vi "graph4.vi"(11 "replay":bool) -> (0 "y":dynamicdata(graph), 3 "x":dynamicdata(graph), 4 "size(s)":i32)   [LabVIEW 2015]
uses:
  G_SEN.vi
  G_LCM.vi
  <vilib>/Analysis/polynomials.llb/1D Polynomial Evaluation (DBL).vi
  G_ALL.vi
  <vilib>/Analysis/NI_AALPro.lvlib
panel:
  out "y 4":dbl[](array[numeric])
  out "x 3":dbl[](array[numeric])
  out "y 3":dbl[](array[numeric])
  out "x 2":dbl[](array[numeric])
  in  "y 2":dbl=3.9000000000000004 format="%#_13g"
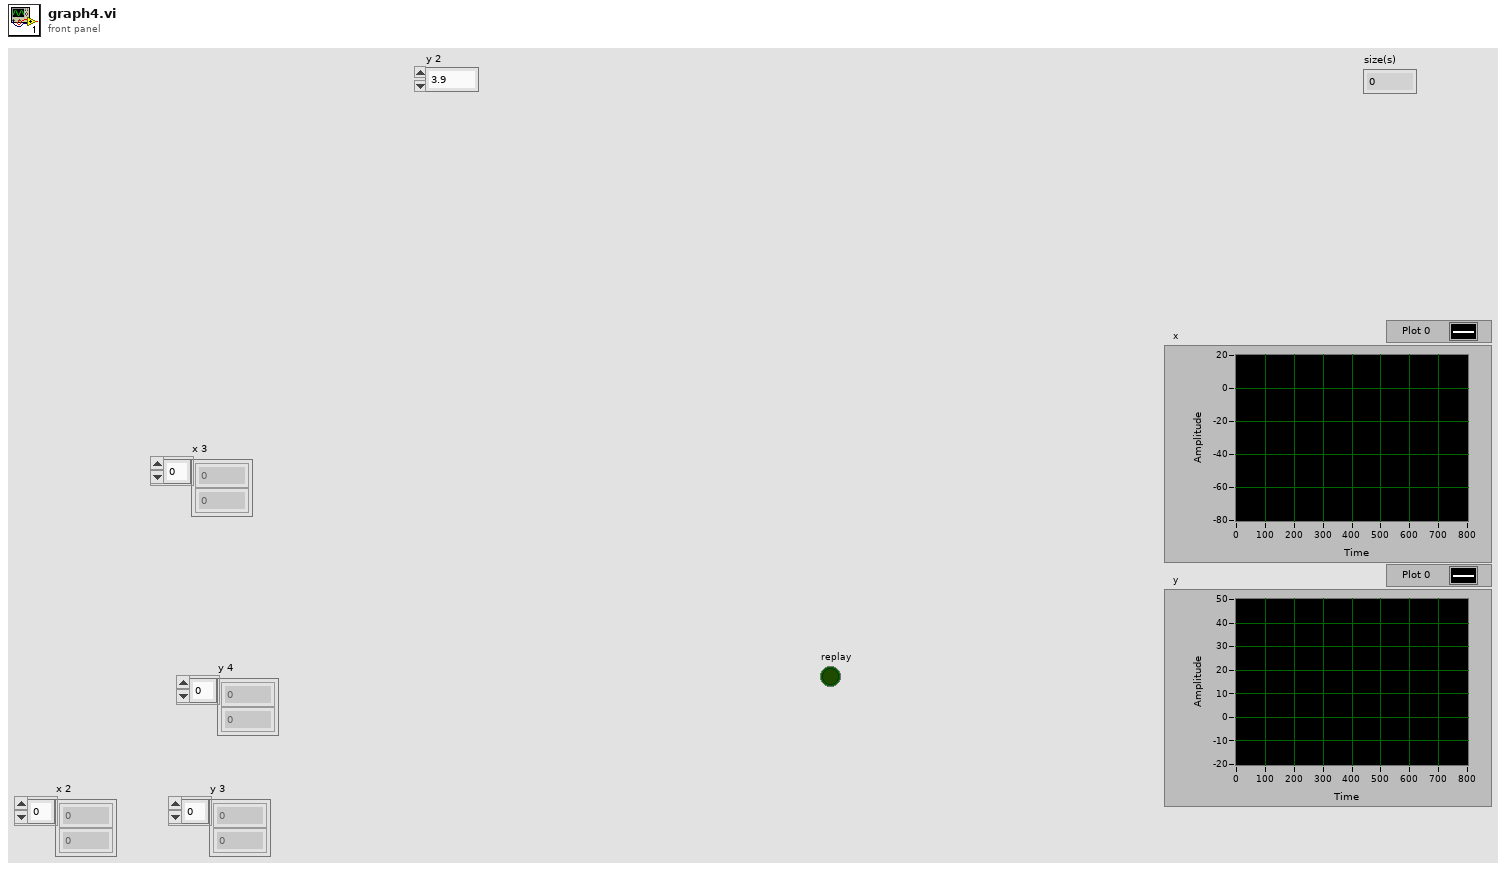
[diagram p1: front panel]
types:
  T1 = cluster{"Steer_input":dbl, "Steer_output":dbl, "VS_des":dbl, "VS_can":dbl, "heading":dbl, "auto":bool, "run":bool, "x":dbl, "y":dbl, "slam_y":dbl, "slam_x":dbl, "slam_heading":dbl}
  T2 = cluster{"C_Wheel base":dbl, "ratio_steer":dbl, "Overall width":dbl, "af":dbl, "turn radius":dbl, "eval":dbl, "ap":dbl, "an":dbl, "Vmax":dbl, "mu":dbl, "Vlast":dbl}
  T3 = cluster{"delta":bool, "Rotational position":dbl, "Rotational position":dbl}[]
  T4 = cluster{"element":sgl, "element":sgl, "element":sgl, "element":sgl, "element":sgl}[]
  T5 = cluster{"hash":i64, "sys time":i64, "stopline_exist":bool, "stopline_distance":dbl}
  T6 = cluster{"hash":i64, "sys time":i64, "size":i64, "x":dbl[], "y":dbl[], "point_flag":i32[]}
  T7 = cluster{"hash":i64, "sys time":i64, "time":dbl, "x":dbl, "y":dbl, "h":dbl, "numSV":i32, "postype":i32, "lag":i32, "hordev":dbl, "lat":dbl, "lon":dbl, "hgt":dbl, "map_idx":i32}
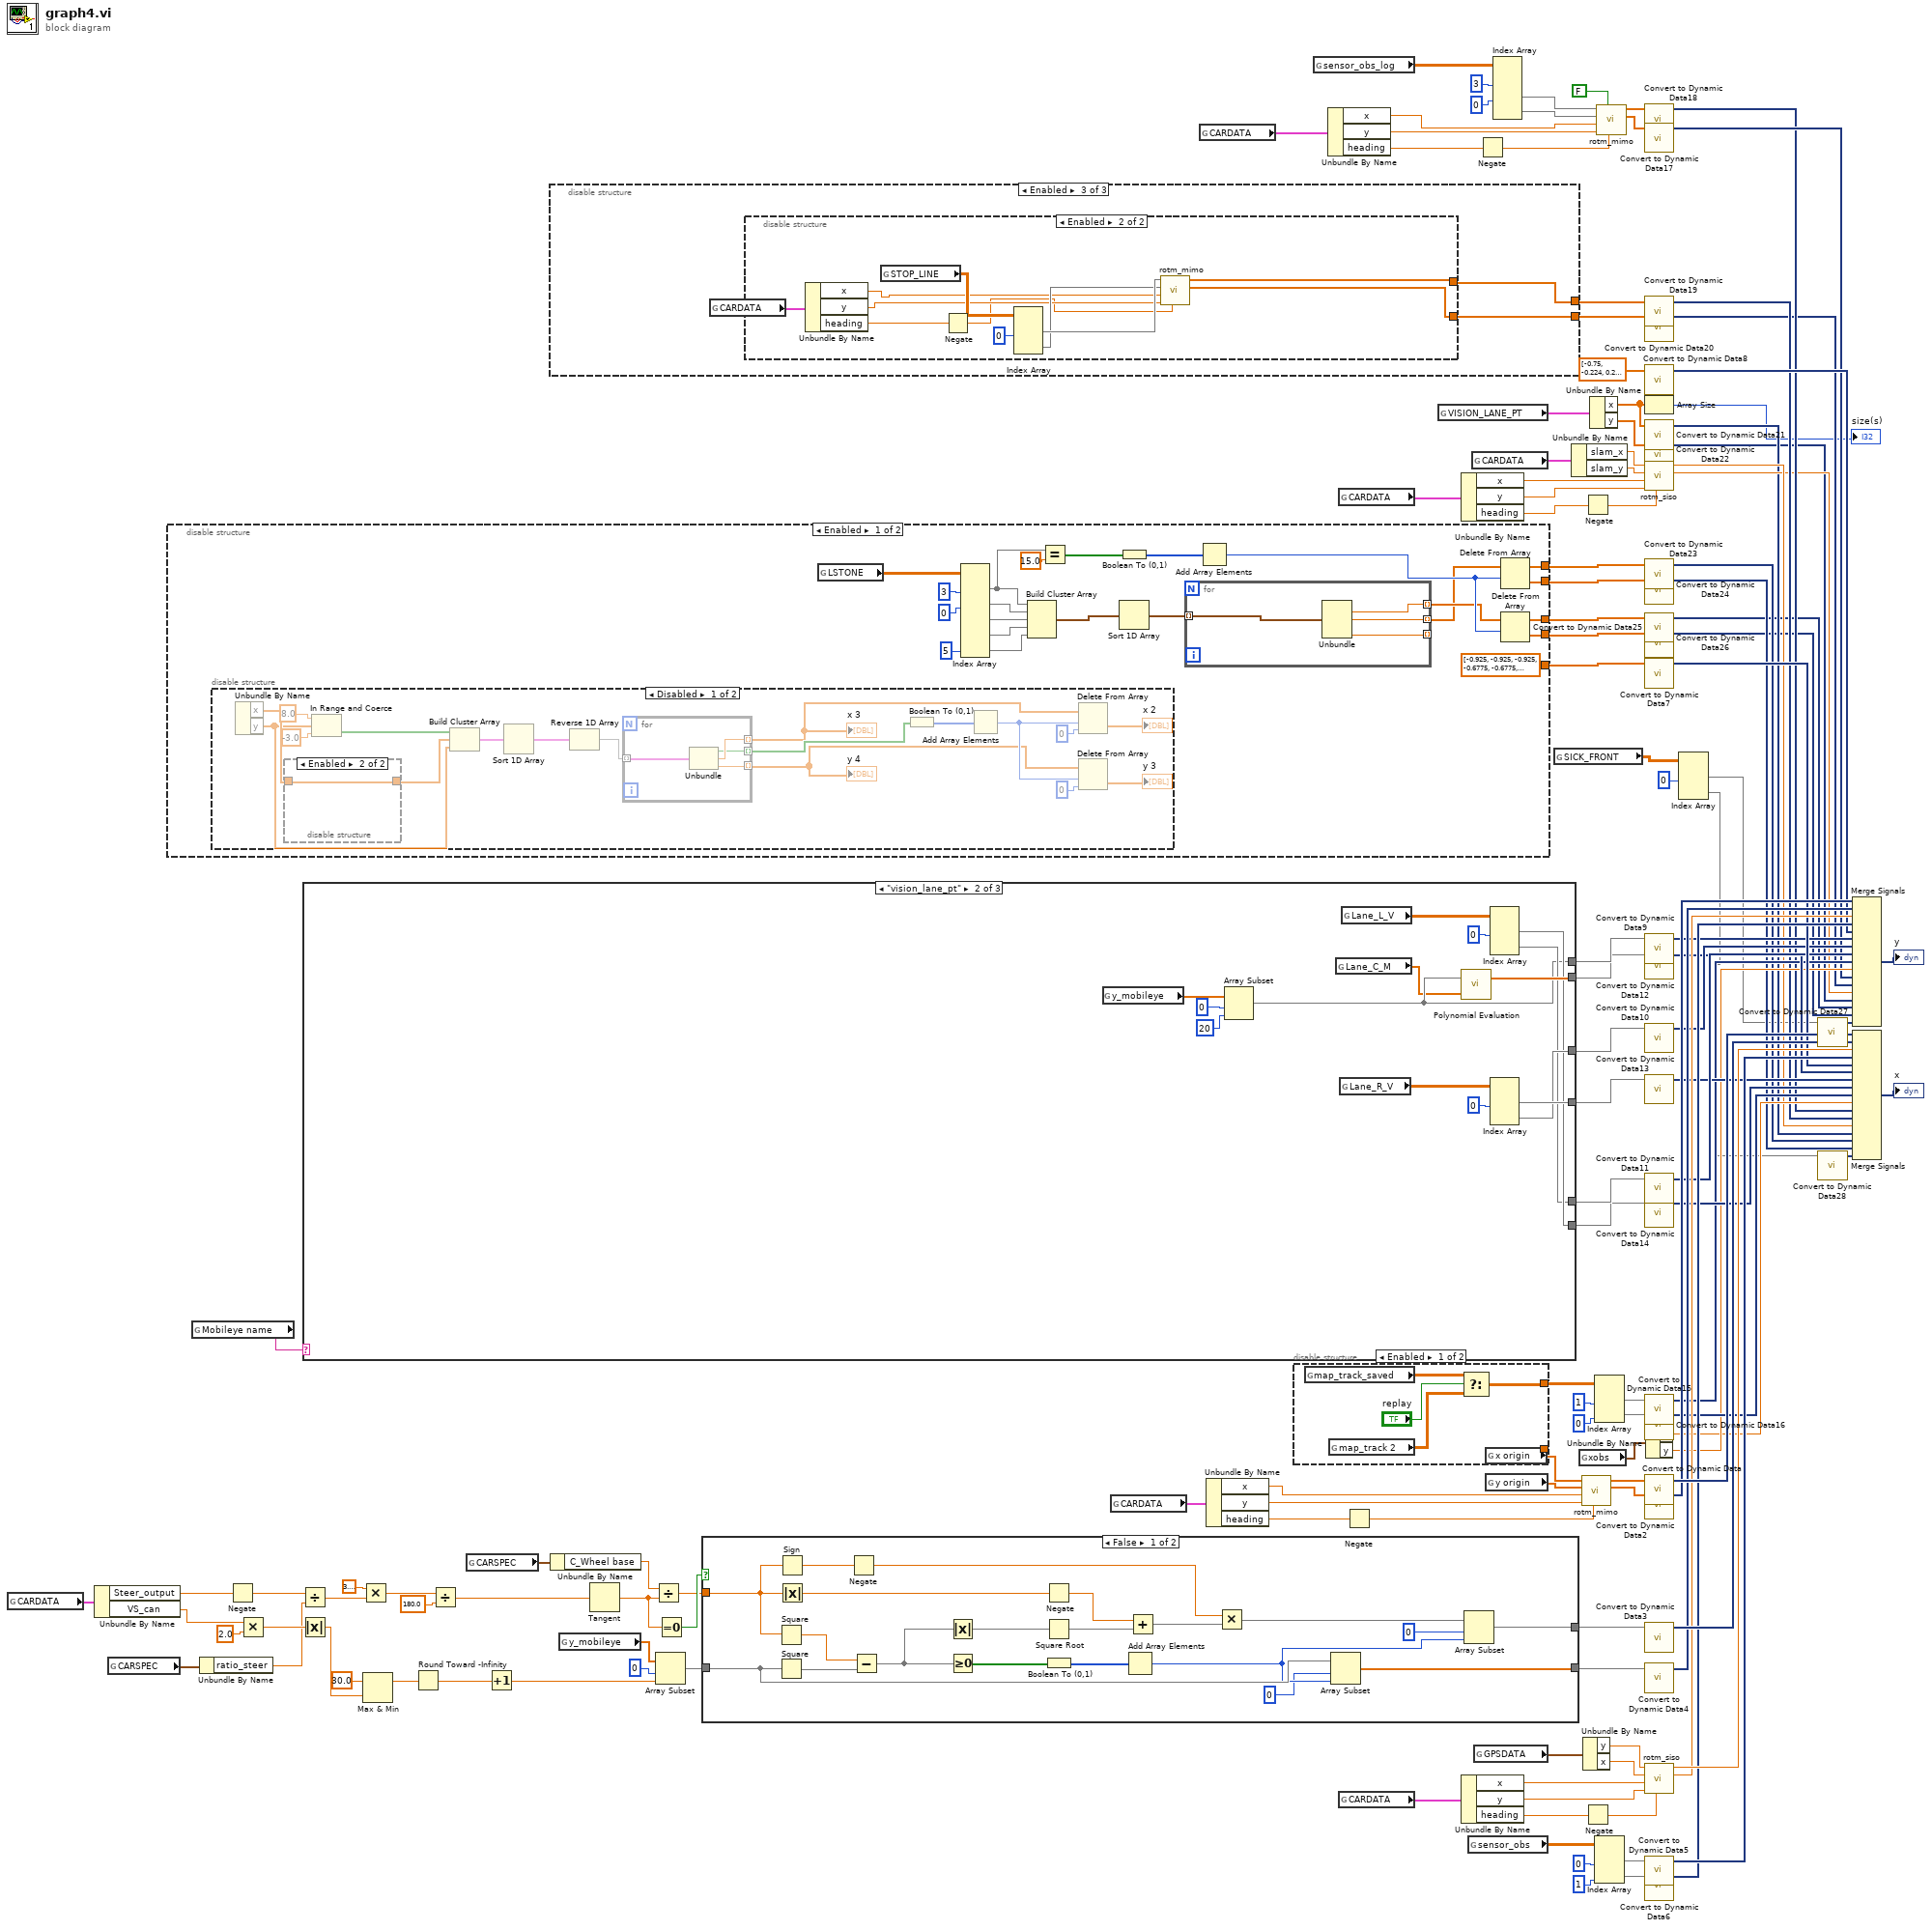
[diagram p0: block diagram]
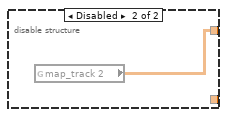
[diagram p2: hidden frame]
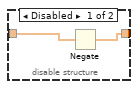
[diagram p3: hidden frame]
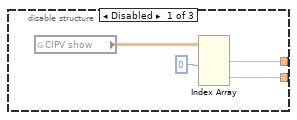
[diagram p6: hidden frame]
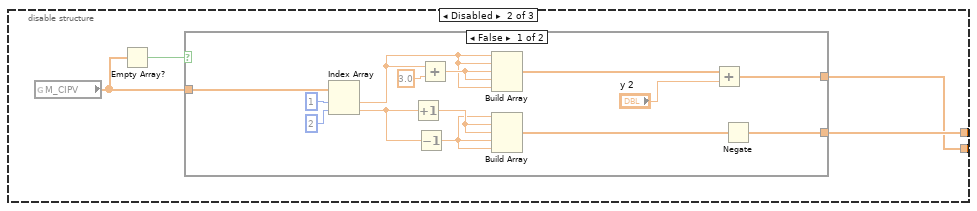
[diagram p7: hidden frame]
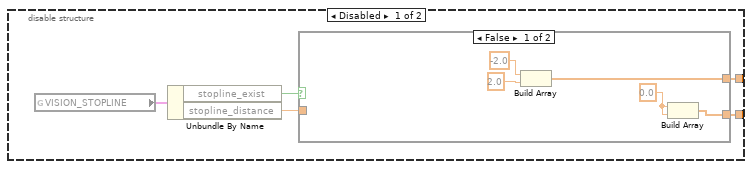
[diagram p9: hidden frame]
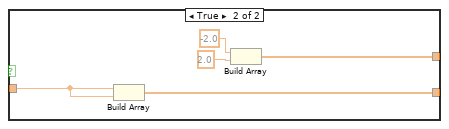
[diagram p10: hidden frame]
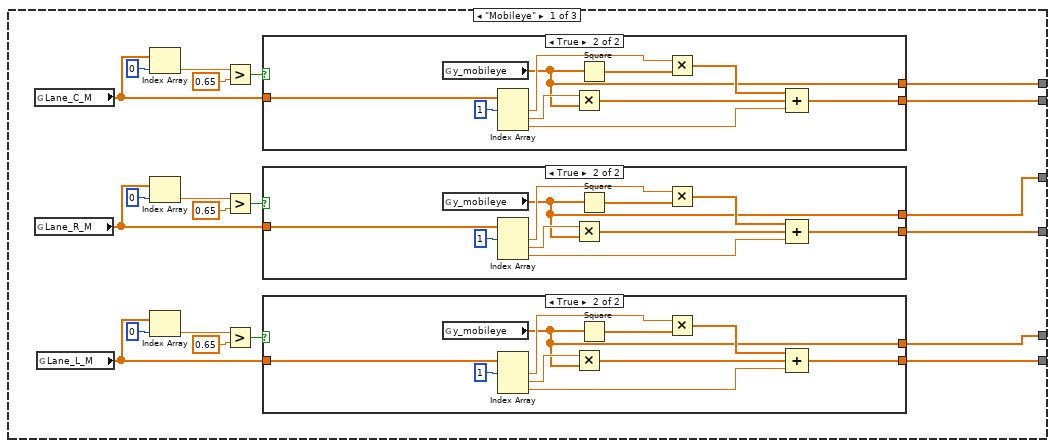
[diagram p11: hidden frame]
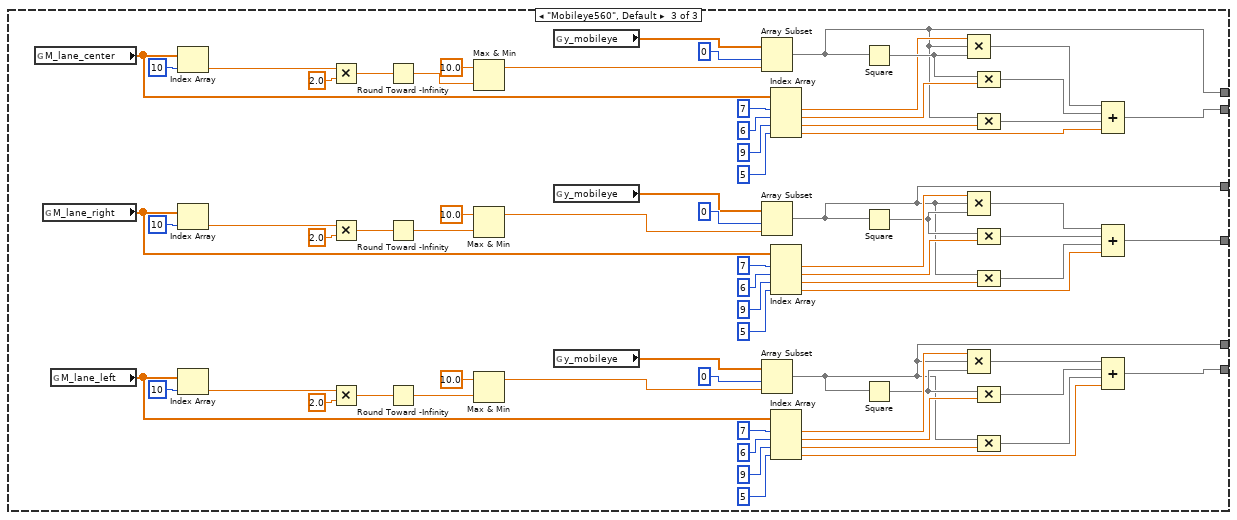
[diagram p15: hidden frame]
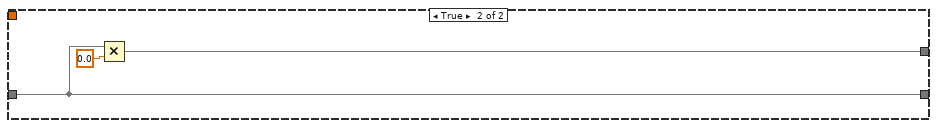
[diagram p16: hidden frame]
diagram:
  n1 = global read "G_ALL.vi" "CARDATA"() -> (w42:T1)
  n2 = Unbundle By Name(w42) -> ("Steer_output"=w86:dbl, "VS_can"=w113:dbl)
  n3 = global read "G_ALL.vi" "CARSPEC"() -> (w33:T2)
  n4 = disable-structure shown="Enabled" {
    disable-tunnel: [dbl[] [-0.925, -0.925, -0.925, -0.6775, -0.6775, -0.925, -0.925, -0.925, -0.925, -0.6775, -0.6775, -0.925, -0.925, -0.925, 0.9025, 0.9025, 0.9025, 0.6775, 0.6775, 0.9025, 0.9025, 0.9025, 0.9025, 0.6775, 0.6775, 0.9025, 0.9025, 0.9025, -0.925] ("car_x") _] -> w88
    disable-tunnel: [w144 _] -> w14
    disable-tunnel: [w143 _] -> w12
    disable-tunnel: [w142 _] -> w10
    disable-tunnel: [w141 _] -> w8
    frame Enabled {
      n5 = disable-structure shown="Disabled" {
        frame Disabled {
          n6 = Unbundle By Name() -> ("x"=w175:dbl[], "y"=w169:dbl[])  [unwired: 1 in]
          n7 = disable-structure shown="Enabled" {
            disable-tunnel: w175 -> [w178 w179]
            disable-tunnel: [w177 w179] -> w176
            frame Disabled {
              n8 = Negate(x=w178) -> (-x=w177:dbl[])
            }
            frame Enabled {
            }
          }
          n9 = In Range and Coerce(upper limit=8.0 ("delta"), x=w169, lower limit=-3.0) -> (In Range?=w167:bool[])  [unwired: 1 out]
          n10 = Build Cluster Array(w167, w176, w169) -> (w165:T3)
          n11 = Sort 1D Array(array=w165) -> (sorted array=w166:T3)
          n12 = Reverse 1D Array(array=w166) -> (reversed array=w162:T3)
          n13 = for {
            tunnel: w162 -> [w183] mode=indexing
            tunnel: [w182] -> w160 mode=indexing
            tunnel: [w181] -> w159 mode=indexing
            tunnel: [w180] -> w170 mode=indexing
            n14 = Unbundle(w183) -> ("delta"=w180:bool, "Rotational position"=w182:dbl, "Rotational position"=w181:dbl)
          }
          "x 3" <- w160
          "y 4" <- w159
          n15 = Boolean To (0,1)(Boolean=w170) -> (0, 1=w163:i16[])
          n16 = Add Array Elements(numeric array=w163) -> (sum=w171:i16)
          n17 = Delete From Array(array=w160, length=w171, index=0) -> (deleted portion=→"x 2":dbl[])  [unwired: 1 out]
          n18 = Delete From Array(array=w159, length=w171, index=0) -> (deleted portion=→"y 3":dbl[])  [unwired: 1 out]
        }
        frame Enabled {
        }
      }
      n19 = global read "G_SEN.vi" "LSTONE"() -> (w157:sgl[][])
      n20 = Index Array(array=w157, index (col) #1=3 ("disabled index (col)"), index (col) #2=0 ("index (col)"), index (col) #5=5 ("index (col)")) -> (element #1=w150:sgl[], element #2=w154:sgl[], element #3=w153:sgl[], element #4=w152:sgl[], element #5=w139:sgl[])  [unwired: 7 in]
      n21 = Build Cluster Array(w150, w154, w153, w152, w139) -> (w151:T4)
      n22 = Equal?(x=w150, y=15.0) -> (x = y?=w148:bool[])
      n23 = Boolean To (0,1)(Boolean=w148) -> (0, 1=w147:i16[])
      n24 = Sort 1D Array(array=w151) -> (sorted array=w146:T4)
      n25 = for {
        tunnel: w146 -> [w187] mode=indexing
        tunnel: [w186] -> w138 mode=indexing
        tunnel: [w185] -> w137 mode=indexing
        tunnel: [w184] -> _ mode=indexing
        n26 = Unbundle(w187) -> ("element"=w186:sgl, "element"=w185:sgl, "element"=w184:sgl)  [unwired: 2 out]
      }
      n27 = Add Array Elements(numeric array=w147) -> (sum=w145:i16)
      n28 = Delete From Array(array=w137, length=w145) -> (deleted portion=w143:sgl[], array with subset deleted=w144:sgl[])  [unwired: 1 in]
      n29 = Delete From Array(array=w138, length=w145) -> (deleted portion=w141:sgl[], array with subset deleted=w142:sgl[])  [unwired: 1 in]
    }
    frame Disabled {
    }
  }
  n30 = global read "G_LCM.vi" "Mobileye name"() -> (w82:string)
  n31 = Unbundle By Name(w33) -> ("ratio_steer"=w32:dbl)
  n32 = Negate(x=w86) -> (-x=w85:dbl)
  n33 = Multiply(x=w113, y=2.0) -> (x*y=w118:dbl)
  n34 = Divide(x=w85, y=w32) -> (x/y=w128:dbl)
  n35 = Absolute Value(x=w118) -> (abs(x)=w119:dbl)
  n36 = case shown="\"vision_lane_pt\"" w82 {
    tunnel: [w203 w240 w258] -> w81
    tunnel: [w196 w245 w257] -> w79
    tunnel: [w189 w241 w256] -> w77
    tunnel: [w202 w252 w255] -> w75
    tunnel: [w195 w246 w254] -> w73
    tunnel: [w188 w242 w253] -> w71
    frame "Mobileye" {
      n37 = global read "G_SEN.vi" "Lane_C_M"() -> (w207:dbl[])
      n38 = global read "G_SEN.vi" "Lane_R_M"() -> (w198:dbl[])
      n39 = global read "G_SEN.vi" "Lane_L_M"() -> (w193:dbl[])
      n40 = Index Array(array=w207, index=0) -> (element=w205:dbl)
      n41 = Index Array(array=w198, index=0) -> (element=w200:dbl)
      n42 = Index Array(array=w193, index=0) -> (element=w191:dbl)
      n43 = Greater?(x=w205, y=0.65) -> (0:w206:bool)
      n44 = Greater?(x=w200, y=0.65) -> (0:w199:bool)
      n45 = Greater?(x=w191, y=0.65) -> (0:w192:bool)
      n46 = case shown="True" w206 {
        tunnel: w207 -> [_ w230]
        tunnel: [_ w231] -> w202
        tunnel: [_ w229] -> w203
        frame False {
        }
        frame True {
          n47 = global read "G_SEN.vi" "y_mobileye"() -> (w229:dbl[])
          n48 = Index Array(array=w230, index #1=1 ("index")) -> (element #1=w236:dbl, element #2=w235:dbl, element #3=w232:dbl)  [unwired: 2 in]
          n49 = Multiply(x=w235, y=w229) -> (x*y=w233:dbl[])
          n50 = Square(x=w229) -> (x^2=w237:dbl[])
          n51 = Multiply(x=w236, y=w237) -> (x*y=w234:dbl[])
          n52 = Compound Arithmetic op=ADD(w234, w233, w232) -> (w231:dbl[])
        }
      }
      n53 = case shown="True" w199 {
        tunnel: w198 -> [_ w220]
        tunnel: [_ w221] -> w195
        tunnel: [_ w219] -> w196
        frame False {
        }
        frame True {
          n54 = global read "G_SEN.vi" "y_mobileye"() -> (w219:dbl[])
          n55 = Index Array(array=w220, index #1=1 ("index")) -> (element #1=w226:dbl, element #2=w225:dbl, element #3=w222:dbl)  [unwired: 2 in]
          n56 = Multiply(x=w225, y=w219) -> (x*y=w223:dbl[])
          n57 = Square(x=w219) -> (x^2=w227:dbl[])
          n58 = Multiply(x=w226, y=w227) -> (x*y=w224:dbl[])
          n59 = Compound Arithmetic op=ADD(w224, w223, w222) -> (w221:dbl[])
        }
      }
      n60 = case shown="True" w192 {
        tunnel: w193 -> [_ w210]
        tunnel: [_ w211] -> w188
        tunnel: [_ w209] -> w189
        frame False {
        }
        frame True {
          n61 = global read "G_SEN.vi" "y_mobileye"() -> (w209:dbl[])
          n62 = Index Array(array=w210, index #1=1 ("index")) -> (element #1=w216:dbl, element #2=w215:dbl, element #3=w212:dbl)  [unwired: 2 in]
          n63 = Multiply(x=w215, y=w209) -> (x*y=w213:dbl[])
          n64 = Square(x=w209) -> (x^2=w217:dbl[])
          n65 = Multiply(x=w216, y=w217) -> (x*y=w214:dbl[])
          n66 = Compound Arithmetic op=ADD(w214, w213, w212) -> (w211:dbl[])
        }
      }
    }
    frame "vision_lane_pt" {
      n67 = global read "G_SEN.vi" "y_mobileye"() -> (w251:dbl[])
      n68 = Array Subset(array=w251, index=0, length=20) -> (w240:dbl[])
      n69 = global read "G_SEN.vi" "Lane_C_M"() -> (w239:dbl[])
      n70 = global read "G_SEN.vi" "Lane_R_V"() -> (w248:dbl[][])
      n71 = global read "G_SEN.vi" "Lane_L_V"() -> (w243:dbl[][])
      n72 = call-poly <vilib>:"Polynomial Evaluation.vi"("P(x)"=w239, "A"=w240) -> ("P(A)"=w252:dbl[])  [unwired: 1 out]
      n73 = Index Array(array=w243, index (col) #1=0 ("disabled index (col)")) -> (element #1=w242:dbl[], element #2=w241:dbl[])  [unwired: 3 in]
      n74 = Index Array(array=w248, index (col) #1=0 ("disabled index (col)")) -> (element #1=w246:dbl[], element #2=w245:dbl[])  [unwired: 3 in]
    }
    frame "Mobileye560", Default {
      n75 = global read "G_SEN.vi" "M_lane_center"() -> (w265:dbl[])
      n76 = global read "G_SEN.vi" "M_lane_right"() -> (w264:dbl[])
      n77 = global read "G_SEN.vi" "M_lane_left"() -> (w263:dbl[])
      n78 = Index Array(array=w265, index=10) -> (element=w271:dbl)
      n79 = Index Array(array=w264, index=10) -> (element=w300:dbl)
      n80 = Index Array(array=w263, index=10) -> (element=w293:dbl)
      n81 = Multiply(x=w271, y=2.0) -> (x*y=w282:dbl)
      n82 = Multiply(x=w300, y=2.0) -> (x*y=w299:dbl)
      n83 = Multiply(x=w293, y=2.0) -> (x*y=w294:dbl)
      n84 = Round Toward -Infinity(1:w282) -> (0:w268:dbl)
      n85 = Round Toward -Infinity(1:w299) -> (0:w291:dbl)
      n86 = Round Toward -Infinity(1:w294) -> (0:w287:dbl)
      n87 = Max & Min(x=10.0, y=w268) -> (max(x,y)=w285:dbl)  [unwired: 1 out]
      n88 = Max & Min(x=10.0, y=w291) -> (max(x,y)=w289:dbl)  [unwired: 1 out]
      n89 = Max & Min(x=10.0, y=w287) -> (max(x,y)=w286:dbl)  [unwired: 1 out]
      n90 = global read "G_SEN.vi" "y_mobileye"() -> (w259:dbl[])
      n91 = global read "G_SEN.vi" "y_mobileye"() -> (w261:dbl[])
      n92 = global read "G_SEN.vi" "y_mobileye"() -> (w260:dbl[])
      n93 = Array Subset(array=w259, index=0, length=w285) -> (w258:dbl[])
      n94 = Array Subset(array=w261, index=0, length=w289) -> (w257:dbl[])
      n95 = Array Subset(array=w260, index=0, length=w286) -> (w256:dbl[])
      n96 = Index Array(array=w265, index #1=7 ("index"), index #2=6 ("index"), index #3=9 ("index"), index #4=5 ("index")) -> (element #1=w266:dbl, element #2=w279:dbl, element #3=w277:dbl, element #4=w284:dbl)
      n97 = Index Array(array=w264, index #1=7 ("index"), index #2=6 ("index"), index #3=9 ("index"), index #4=5 ("index")) -> (element #1=w323:dbl, element #2=w321:dbl, element #3=w319:dbl, element #4=w315:dbl)
      n98 = Index Array(array=w263, index #1=7 ("index"), index #2=6 ("index"), index #3=9 ("index"), index #4=5 ("index")) -> (element #1=w305:dbl, element #2=w307:dbl, element #3=w309:dbl, element #4=w313:dbl)
      n99 = Square(x=w258) -> (x^2=w273:dbl[])
      n100 = Square(x=w257) -> (x^2=w302:dbl[])
      n101 = Square(x=w256) -> (x^2=w303:dbl[])
      n102 = Compound Arithmetic op=MULTIPLY(w266, w258, w273) -> (w276:dbl[])
      n103 = Compound Arithmetic op=MULTIPLY(w323, w257, w302) -> (w318:dbl[])
      n104 = Compound Arithmetic op=MULTIPLY(w305, w256, w303) -> (w310:dbl[])
      n105 = Compound Arithmetic op=MULTIPLY(w273, w279) -> (w275:dbl[])
      n106 = Compound Arithmetic op=MULTIPLY(w258, w277) -> (w274:dbl[])
      n107 = Compound Arithmetic op=MULTIPLY(w302, w321) -> (w317:dbl[])
      n108 = Compound Arithmetic op=MULTIPLY(w257, w319) -> (w316:dbl[])
      n109 = Compound Arithmetic op=MULTIPLY(w303, w307) -> (w311:dbl[])
      n110 = Compound Arithmetic op=MULTIPLY(w256, w309) -> (w312:dbl[])
      n111 = Compound Arithmetic op=ADD(w276, w275, w274, w284) -> (w255:dbl[])
      n112 = Compound Arithmetic op=ADD(w318, w317, w316, w315) -> (w254:dbl[])
      n113 = Compound Arithmetic op=ADD(w310, w311, w312, w313) -> (w253:dbl[])
    }
  }
  n114 = Multiply(x=3.141592653589793, y=w128) -> (x*y=w125:dbl)
  n115 = Max & Min(x=30.0, y=w119) -> (max(x,y)=w120:dbl)  [unwired: 1 out]
  n116 = Round Toward -Infinity(1:w120) -> (0:w115:dbl)
  n117 = Divide(x=w125, y=180.0) -> (x/y=w127:dbl)
  n118 = global read "G_ALL.vi" "CARSPEC"() -> (w34:T2)
  n119 = Increment(x=w115) -> (x+1=w117:dbl)
  n120 = disable-structure shown="Enabled" {
    disable-tunnel: [w326 w332 w348] -> w47
    disable-tunnel: [w325 w331 w347] -> w45
    frame Disabled {
      n121 = global read "G_SEN.vi" "CIPV show"() -> (w328:dbl[][])
      n122 = Index Array(array=w328, index (col) #1=0 ("disabled index (col)")) -> (element #1=w326:dbl[], element #2=w325:dbl[])  [unwired: 3 in]
    }
    frame Disabled {
      n123 = global read "G_SEN.vi" "M_CIPV"() -> (w329:dbl[])
      n124 = Empty Array?(array=w329) -> (empty?=w330:bool)
      n125 = case shown="False" w330 {
        tunnel: [w333 _] -> w332
        tunnel: [w336 _] -> w331
        tunnel: w329 -> [w338 _]
        frame False {
          n126 = Index Array(array=w338, index #1=1 ("index"), index #2=2 ("index")) -> (element #1=w339:dbl, element #2=w343:dbl)
          n127 = Increment(x=w343) -> (x+1=w344:dbl)
          n128 = Decrement(x=w343) -> (x-1=w342:dbl)
          n129 = Add(x=w339, y=3.0) -> (x+y=w340:dbl)
          n130 = Build Array(w339, w339, w340, w340, w339) -> (w337:dbl[])
          n131 = Build Array(w342, w344, w344, w342, w342) -> (w334:dbl[])
          n132 = Add(x=w337, y="y 2") -> (x+y=w336:dbl[])
          n133 = Negate(x=w334) -> (-x=w333:dbl[])
        }
        frame True {
        }
      }
    }
    frame Enabled {
      n134 = disable-structure shown="Enabled" {
        disable-tunnel: [w350 w365] -> w348
        disable-tunnel: [w349 w364] -> w347
        frame Disabled {
          n135 = global read "G_LCM.vi" "VISION_STOPLINE"() -> (w351:T5)
          n136 = Unbundle By Name(w351) -> ("stopline_exist"=w352:bool, "stopline_distance"=w353:dbl)
          n137 = case shown="False" w352 {
            tunnel: w353 -> [_ w360]
            tunnel: [w356 w361] -> w350
            tunnel: [w355 w359] -> w349
            frame False {
              w354 = 0.0 ("element")
              n138 = Build Array(-2.0 ("element"), 2.0 ("element")) -> (w356:dbl[])
              n139 = Build Array(w354, w354) -> (w355:dbl[])
            }
            frame True {
              n140 = Build Array(w360, w360) -> (w359:dbl[])
              n141 = Build Array(-2.0 ("element"), 2.0 ("element")) -> (w361:dbl[])
            }
          }
        }
        frame Enabled {
          n142 = global read "G_ALL.vi" "CARDATA"() -> (w369:T1)
          n143 = Unbundle By Name(w369) -> ("x"=w368:dbl, "y"=w367:dbl, "heading"=w370:dbl)
          n144 = global read "G_ALL.vi" "STOP_LINE"() -> (w374:dbl[][])
          n145 = Negate(x=w370) -> (-x=w366:dbl)
          n146 = Index Array(array=w374, index (col) #1=0 ("disabled index (col)")) -> (element #1=w372:dbl[], element #2=w371:dbl[])  [unwired: 3 in]
          n147 = call "rotm_mimo.vi"("angle[rad]"=w366, "y0"=w367, "x0"=w368, "y"=w371, "x"=w372) -> ("Y"=w364:dbl[], "X"=w365:dbl[])  [unwired: 3 in, 2 out]
        }
      }
    }
  }
  n148 = Unbundle By Name(w34) -> ("C_Wheel base"=w31:dbl)
  n149 = global read "G_SEN.vi" "y_mobileye"() -> (w112:dbl[])
  n150 = Tangent(1:w127) -> (0:w123:dbl)
  n151 = Divide(x=w31, y=w123) -> (x/y=w111:dbl)
  n152 = Array Subset(array=w112, index=0, length=w117) -> (w110:dbl[])
  n153 = Equal To 0?(x=w123) -> (x = 0?=w122:bool)
  n154 = case shown="False" w122 {
    tunnel: w111 -> [w390 _]
    tunnel: [w380 w395] -> w109
    tunnel: w110 -> [w378 w397]
    tunnel: [w376 w397] -> w107
    frame False {
      n155 = Square(x=w390) -> (x^2=w394:dbl)
      n156 = Square(x=w378) -> (x^2=w386:dbl[])
      n157 = Sign(1:w390) -> (0:w389:dbl)
      n158 = Absolute Value(x=w390) -> (abs(x)=w392:dbl)
      n159 = Negate(x=w389) -> (-x=w388:dbl)
      n160 = Subtract(x=w394, y=w386) -> (x-y=w384:dbl[])
      n161 = Absolute Value(x=w384) -> (abs(x)=w393:dbl[])
      n162 = Greater Or Equal To 0?(x=w384) -> (x >= 0?=w383:bool[])
      n163 = Negate(x=w392) -> (-x=w391:dbl)
      n164 = Square Root(x=w393) -> (sqrt(x)=w385:dbl[])
      n165 = Boolean To (0,1)(Boolean=w383) -> (0, 1=w382:i16[])
      n166 = Add Array Elements(numeric array=w382) -> (sum=w377:i16)
      n167 = Add(x=w391, y=w385) -> (x+y=w387:dbl[])
      n168 = Multiply(x=w388, y=w387) -> (x*y=w381:dbl[])
      n169 = Array Subset(array=w378, index=0, length=w377) -> (w376:dbl[])
      n170 = Array Subset(array=w381, index=0, length=w377) -> (w380:dbl[])
    }
    frame True {
      n171 = Multiply(x=w397, y=0.0) -> (x*y=w395:dbl[])
    }
  }
  n172 = global read "G_ALL.vi" "CARDATA"() -> (w41:T1)
  n173 = global read "G_ALL.vi" "CARDATA"() -> (w39:T1)
  n174 = Unbundle By Name(w41) -> ("x"=w135:dbl, "y"=w134:dbl, "heading"=w136:dbl)
  n175 = disable-structure shown="Enabled" {
    disable-tunnel: [w401 w403] -> w43
    disable-tunnel: [w400 _] -> w37
    frame Enabled {
      n176 = global read "G_ALL.vi" "map_track_saved"() -> (w399:dbl[][])
      n177 = global read "G_ALL.vi" "map_track 2"() -> (w398:dbl[][])
      n178 = Select(t=w399, s="replay", f=w398) -> (s? t:f=w401:dbl[][])
      n179 = global read "G_ALL.vi" "x origin"() -> (w400:dbl[])
    }
    frame Disabled {
      n180 = global read "G_ALL.vi" "map_track 2"() -> (w403:dbl[][])
    }
  }
  n181 = global read "G_SEN.vi" "sensor_obs_log"() -> (w52:dbl[][])
  n182 = Unbundle By Name(w39) -> ("x"=w57:dbl, "y"=w58:dbl, "heading"=w56:dbl)
  n183 = global read "G_ALL.vi" "CARDATA"() -> (w30:T1)
  n184 = global read "G_ALL.vi" "CARDATA"() -> (w40:T1)
  n185 = Negate(x=w136) -> (-x=w133:dbl)
  n186 = global read "G_LCM.vi" "VISION_LANE_PT"() -> (w21:T6)
  n187 = Unbundle By Name(w30) -> ("x"=w25:dbl, "y"=w26:dbl, "heading"=w24:dbl)
  n188 = Unbundle By Name(w40) -> ("x"=w104:dbl, "y"=w103:dbl, "heading"=w105:dbl)
  n189 = global read "G_SEN.vi" "sensor_obs"() -> (w95:dbl[][])
  n190 = global read "G_ALL.vi" "CARDATA"() -> (w15:T1)
  n191 = global read "G_ALL.vi" "GPSDATA"() -> (w38:T7)
  n192 = Negate(x=w56) -> (-x=w59:dbl)
  n193 = global read "G_ALL.vi" "y origin"() -> (w36:dbl[])
  n194 = Index Array(array=w52, index (col) #1=3 ("disabled index (col)"), index (col) #2=0 ("disabled index (col)")) -> (element #2=w55:dbl[], element #3=w54:dbl[])  [unwired: 4 in, 1 out]
  n195 = global read "G_SEN.vi" "SICK_FRONT"() -> (w6:sgl[][])
  n196 = Unbundle By Name(w15) -> ("slam_x"=w28:dbl, "slam_y"=w29:dbl)
  n197 = global read "G_ALL.vi" "xobs"() -> (w35:cluster{"idx":i32, "x":dbl, "y":dbl, "h":dbl})
  n198 = call "rotm_mimo.vi"("angle[rad]"=w133, "y0"=w134, "x0"=w135, "y"=w36, "x"=w37) -> ("Y"=w130:dbl[], "X"=w132:dbl[])  [unwired: 3 in, 2 out]
  n199 = Unbundle By Name(w38) -> ("y"=w101:dbl, "x"=w100:dbl)
  n200 = Negate(x=w24) -> (-x=w27:dbl)
  n201 = Negate(x=w105) -> (-x=w102:dbl)
  n202 = Unbundle By Name(w21) -> ("x"=w17:dbl[], "y"=w18:dbl[])
  n203 = Index Array(array=w43, index (col) #1=1 ("disabled index (col)"), index (col) #2=0 ("index (col)")) -> (element #1=w68:dbl[], element #2=w66:dbl[])  [unwired: 2 in]
  n204 = Index Array(array=w95, index (col) #1=0 ("disabled index (col)"), index (col) #2=1 ("index (col)")) -> (element #1=w94:dbl[], element #2=w92:dbl[])  [unwired: 2 in]
  n205 = call "rotm_mimo.vi"("angle[rad]"=w59, "reverse"=FALSE, "y0"=w58, "x0"=w57, "y"=w54, "x"=w55) -> ("Y"=w51:dbl[], "X"=w49:dbl[])  [unwired: 2 in, 2 out]
  n206 = call "Convert to Dynamic Data18"("Array"=w49) -> ("Dynamic Data Type"=w48:dynamicdata)  [unwired: 3 in]
  n207 = call "Convert to Dynamic Data17"("Array"=w51) -> ("Dynamic Data Type"=w50:dynamicdata)  [unwired: 3 in]
  n208 = call "Convert to Dynamic Data19"("Array"=w47) -> ("Dynamic Data Type"=w46:dynamicdata)  [unwired: 3 in]
  n209 = call "Convert to Dynamic Data20"("Array"=w45) -> ("Dynamic Data Type"=w44:dynamicdata)  [unwired: 3 in]
  n210 = call "Convert to Dynamic Data8"("Array"=dbl[] [-0.75, -0.224, 0.224, 0.224, -0.224, -0.224, 0.224, 2.415, 2.885, 2.885, 2.415, 2.415, 2.885, 3.5, 3.5, 2.885, 2.415, 2.415, 2.885, 2.885, 2.415, 0.224, -0.224, -0.224, 0.224, 0.224, -0.224, -0.75, -0.75] ("car_y")) -> ("Dynamic Data Type"=w89:dynamicdata)  [unwired: 3 in]
  n211 = Array Size(array=w17) -> (size(s)=→"size(s)":i32)
  n212 = call "Convert to Dynamic Data21"("Array"=w17) -> ("Dynamic Data Type"=w20:dynamicdata)  [unwired: 3 in]
  n213 = call "Convert to Dynamic Data22"("Array"=w18) -> ("Dynamic Data Type"=w19:dynamicdata)  [unwired: 3 in]
  n214 = call "rotm_siso.vi"("angle[rad]"=w27, "y0"=w26, "x0"=w25, "y"=w29, "x"=w28) -> ("y'"=w22:dbl, "x'"=w23:dbl)  [unwired: 5 in]
  n215 = call "Convert to Dynamic Data23"("Array"=w14) -> ("Dynamic Data Type"=w13:dynamicdata)  [unwired: 3 in]
  n216 = call "Convert to Dynamic Data24"("Array"=w12) -> ("Dynamic Data Type"=w11:dynamicdata)  [unwired: 3 in]
  n217 = call "Convert to Dynamic Data25"("Array"=w10) -> ("Dynamic Data Type"=w9:dynamicdata)  [unwired: 3 in]
  n218 = call "Convert to Dynamic Data26"("Array"=w8) -> ("Dynamic Data Type"=w7:dynamicdata)  [unwired: 3 in]
  n219 = call "Convert to Dynamic Data7"("Array"=w88) -> ("Dynamic Data Type"=w90:dynamicdata)  [unwired: 3 in]
  n220 = call "Convert to Dynamic Data9"("Array"=w81) -> ("Dynamic Data Type"=w80:dynamicdata)  [unwired: 3 in]
  n221 = call "Convert to Dynamic Data12"("Array"=w75) -> ("Dynamic Data Type"=w74:dynamicdata)  [unwired: 3 in]
  n222 = call "Convert to Dynamic Data10"("Array"=w79) -> ("Dynamic Data Type"=w78:dynamicdata)  [unwired: 3 in]
  n223 = call "Convert to Dynamic Data13"("Array"=w73) -> ("Dynamic Data Type"=w72:dynamicdata)  [unwired: 3 in]
  n224 = call "Convert to Dynamic Data11"("Array"=w77) -> ("Dynamic Data Type"=w76:dynamicdata)  [unwired: 3 in]
  n225 = call "Convert to Dynamic Data14"("Array"=w71) -> ("Dynamic Data Type"=w70:dynamicdata)  [unwired: 3 in]
  n226 = call "Convert to Dynamic Data15"("Array"=w68) -> ("Dynamic Data Type"=w67:dynamicdata)  [unwired: 3 in]
  n227 = call "Convert to Dynamic Data16"("Array"=w66) -> ("Dynamic Data Type"=w65:dynamicdata)  [unwired: 3 in]
  n228 = call "Convert to Dynamic Data"("Array"=w132) -> ("Dynamic Data Type"=w131:dynamicdata)  [unwired: 3 in]
  n229 = call "Convert to Dynamic Data2"("Array"=w130) -> ("Dynamic Data Type"=w129:dynamicdata)  [unwired: 3 in]
  n230 = call "Convert to Dynamic Data3"("Array"=w109) -> ("Dynamic Data Type"=w108:dynamicdata)  [unwired: 3 in]
  n231 = call "Convert to Dynamic Data4"("Array"=w107) -> ("Dynamic Data Type"=w106:dynamicdata)  [unwired: 3 in]
  n232 = call "rotm_siso.vi"("angle[rad]"=w102, "y0"=w103, "x0"=w104, "y"=w100, "x"=w101) -> ("y'"=w98:dbl, "x'"=w99:dbl)  [unwired: 5 in]
  n233 = call "Convert to Dynamic Data5"("Array"=w94) -> ("Dynamic Data Type"=w93:dynamicdata)  [unwired: 3 in]
  n234 = call "Convert to Dynamic Data6"("Array"=w92) -> ("Dynamic Data Type"=w91:dynamicdata)  [unwired: 3 in]
  n235 = Unbundle By Name(w35) -> ("x"=w62:dbl, "y"=w63:dbl)
  n236 = Index Array(array=w6, index (col) #1=0 ("disabled index (col)")) -> (element #1=w4:sgl[], element #2=w2:sgl[])  [unwired: 3 in]
  n237 = call "Convert to Dynamic Data27"("Array"=w4) -> ("Dynamic Data Type"=w3:dynamicdata)  [unwired: 3 in]
  n238 = call "Convert to Dynamic Data28"("Array"=w2) -> ("Dynamic Data Type"=w1:dynamicdata)  [unwired: 3 in]
  n239 = Merge Signals(w129, w106, w98, w91, w89, w80, w78, w76, w67, w63, w50, w44, w22, w19, w9, w7, w3) -> (→"y":dynamicdata)
  n240 = Merge Signals(w131, w108, w99, w93, w90, w74, w72, w70, w65, w62, w48, w46, w23, w20, w13, w11, w1) -> (→"x":dynamicdata)
